vi "Main Body.vi"(8 "error in":errorcluster, 10 "File Actor In":refnum<class "File Actor.lvclass">, 11 "Exe Write Main CMD in":refnum<class "Exe Write PAS Wvfm CMD.lvclass">) -> (0 "error out":errorcluster)   [LabVIEW 2018, in "Controller.lvlib" / "Exe Write PAS Wvfm CMD.lvclass"]
uses:
  Exe Write PAS Wvfm CMD.lvclass
  File Actor/File Actor.lvclass
  C:/Program Files (x86)/National Instruments/LabVIEW 2018/vi.lib/MSR Consulting, LLC/General Reuse/SuperActor/SuperActor.lvclass
  <vilib>/MSR Consulting, LLC/General Reuse/Data/Data.lvclass
  <vilib>/MSR Consulting, LLC/General Reuse/SuperActor/SuperActor.lvclass/SuperActor.ctl
  File Actor/File Actor.lvclass/File Actor.ctl
  Exe Write PAS Wvfm CMD.lvclass/Exe Write PAS Wvfm CMD.ctl
  <vilib>/MSR Consulting, LLC/General Reuse/PAS/Data/Main/PAS Data.lvclass
  C:/Program Files (x86)/National Instruments/LabVIEW 2018/vi.lib/MSR Consulting, LLC/General Reuse/Data/Data.lvclass
  <vilib>/MSR Consulting, LLC/General Reuse/SuperActor/Read Log Session.vi
  File Actor/Read File DVR.vi
  <vilib>/MSR Consulting, LLC/General Reuse/Data/Read measTime.vi
  <vilib>/MSR Consulting, LLC/General Reuse/PAS/Data/Main/Read CellData.vi
  <vilib>/MSR Consulting, LLC/General Reuse/PAS/Data/Cell/Read timeData.vi
  <vilib>/MSR Consulting, LLC/General Reuse/PAS/Data/Cell/Read lasDiodeData.vi
  <vilib>/MSR Consulting, LLC/General Reuse/Session APIs/_Session Fwk/Session - Root.lvclass
  <vilib>/MSR Consulting, LLC/General Reuse/PAS/Data/Cell/PAS Cell Data.lvclass
  <vilib>/MSR Consulting, LLC/General Reuse/Session APIs/Session Log/System Log.lvclass
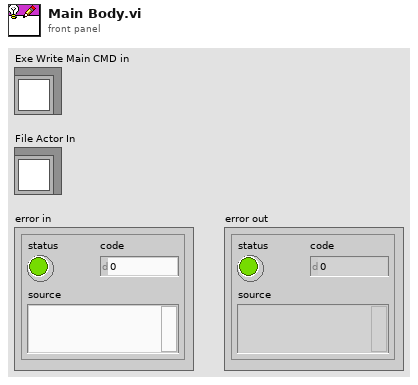
[diagram p1: front panel]
types:
  T1 = typedef "Session - Root.lvclass/Session Handle.ctl" = refnum<data-value>
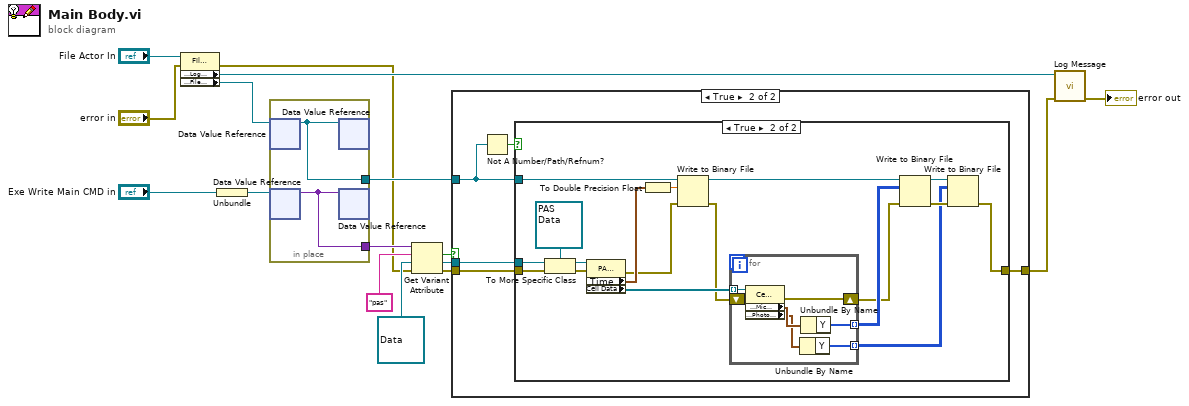
[diagram p0: block diagram]
diagram:
  n1 = property class="File Actor"(reference="File Actor In", error in="error in") -> (error out=w3:errorcluster, "Accessors:Log Session"=w6:T1, "Accessors:File DVR"=w13:refnum<data-value>)  [unwired: 1 out]
  n2 = Unbundle("Exe Write Main CMD in") -> (w15:refnum<data-value>)
  n3 = in-place {
    in-place-border: [w18] -> w7
    in-place-border: [w17] -> w12
    n4 = in-place-dvr #1(w13) -> (w18:refnum<file>)  [unwired: 1 out]
    n5 = in-place-dvr #2(w15) -> (w17:variant)  [unwired: 1 out]
    n6 = in-place-dvr #1(w18) -> ()  [unwired: 2 out]
    n7 = in-place-dvr #2(w17) -> ()  [unwired: 2 out]
  }
  n8 = Get Variant Attribute(Variant=w12, name="pas", default value (empty Variant)=refnum<class "Data.lvclass"> refnum ("Base Data Lib:Data"), error in=w3) -> (found=w9:bool, value=w8:refnum<class "Data.lvclass">, error out=w5:errorcluster)  [unwired: 1 out]
  n9 = case shown="True" w9 {
    tunnel: w8 -> [_ w23]
    tunnel: w7 -> [_ w22]
    tunnel: w5 -> [w19 w21]
    tunnel: [w19 w20] -> w4
    frame False {
    }
    frame True {
      n10 = Not A Number/Path/Refnum?(number/path/refnum=w22) -> (NaN/Path/Refnum?=w24:bool)
      n11 = case shown="True" w24 {
        tunnel: w23 -> [_ w43]
        tunnel: w22 -> [_ w39]
        tunnel: w21 -> [w25 w30]
        tunnel: [w25 w26] -> w20
        frame False {
        }
        frame True {
          n12 = To More Specific Class(target class=refnum<class "PAS Data.lvclass"> refnum ("PAS Library.lvlib:PAS Data"), reference=w43, error in=w30) -> (specific class reference=w41:refnum<class "PAS Data.lvclass">, error out=w40:errorcluster)
          n13 = property class="PAS Data"(reference=w41, error in=w40) -> (error out=w29:errorcluster, "Time"=w38:timestamp, "Cell Data"=w36:refnum<class "PAS Cell Data.lvclass">[])  [unwired: 1 out]
          n14 = To Double Precision Float(number=w38) -> (double precision float=w37:dbl)
          n15 = Write to Binary File(file (use dialog)=w39, data=w37, error in=w29) -> (refnum out=w35:refnum<file>, error out=w28:errorcluster)  [unwired: 3 in, 1 out]
          n16 = for {
            tunnel: w36 -> [w50] mode=indexing
            tunnel: [w48] -> w34 mode=indexing
            tunnel: [w46] -> w31 mode=indexing
            shift-right: [w44] -> w27
            shift-left: w28 -> [w45]
            n17 = property class="Cell Data"(reference=w50, error in=w45) -> (error out=w44:errorcluster, "Accessors:Mic Time"=w49:waveform(i16), "Accessors:Photodiode"=w47:waveform(i16))  [unwired: 1 out]
            n18 = Unbundle By Name(w47) -> ("Y"=w46:i16[])
            n19 = Unbundle By Name(w49) -> ("Y"=w48:i16[])
          }
          n20 = Write to Binary File(file (use dialog)=w35, data=w34, error in=w27) -> (refnum out=w32:refnum<file>, error out=w33:errorcluster)  [unwired: 3 in, 1 out]
          n21 = Write to Binary File(file (use dialog)=w32, data=w31, error in=w33) -> (error out=w26:errorcluster)  [unwired: 3 in, 2 out]
        }
      }
    }
  }
  n22 = call <vilib>:"Log Message.vi"("error in"=w4, "session in"=w6) -> ("error out"=→"error out":errorcluster)  [unwired: 8 in, 1 out]
